vi "IT6333A_Get Resource Name.vi"(8 "error in (no error)":errorcluster, 11 "PowerSupply_IT6333A in":refnum<class "PowerSupply_IT6333A.lvclass">) -> (0 "error out":errorcluster, 2 "Resource Name":string, 3 "PowerSupply_IT6333A out":refnum<class "PowerSupply_IT6333A.lvclass">)   [LabVIEW 2017, in "PowerSupply_IT6333A.lvclass"]
uses:
  PowerSupply_IT6333A.lvclass
  PowerSupply_IT6333A.lvclass/PowerSupply_IT6333A.ctl
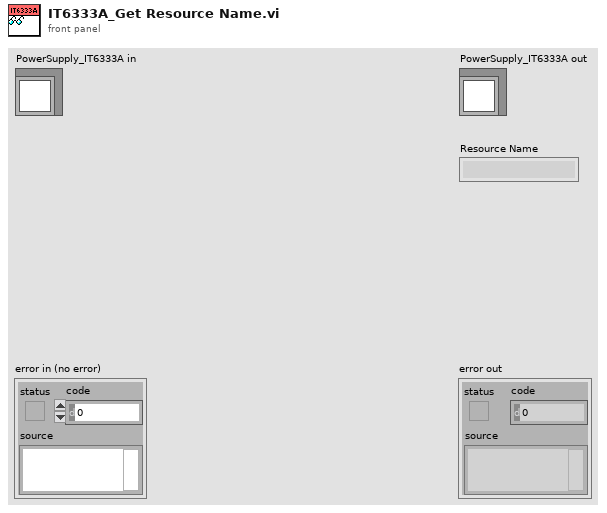
[diagram p1: front panel]
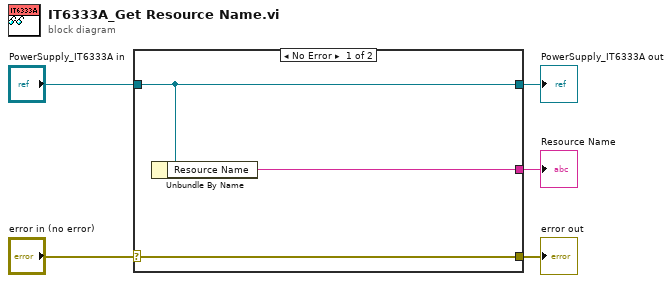
[diagram p0: block diagram]
diagram:
  n1 = case shown="No Error" "error in (no error)" {
    selector: "error in (no error)" -> [w8 w9]
    tunnel: [w8 w9] -> w4
    tunnel: [w7 w10] -> w2
    tunnel: "PowerSupply_IT6333A in" -> [w7 w10]
    tunnel: [w6 _] -> w1
    frame No Error {
      n2 = Unbundle By Name(w7) -> ("Resource Name"=w6:string)
    }
    frame Error {
    }
  }
  "error out" <- w4
  "PowerSupply_IT6333A out" <- w2
  "Resource Name" <- w1
